vi "QMH_Wait_notifier.vi"(8 "error in (no error)":errorcluster) -> (0 "error out":errorcluster, 2 "Payload":variant, 3 "Message":T1)   [LabVIEW 2021, in "Framework_lib.lvlib"]
uses:
  Framework_lib.lvlib
  QMH_producer_enum.ctl
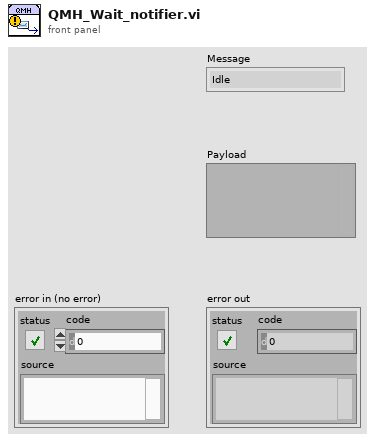
[diagram p1: front panel]
types:
  T1 = typedef "Framework_lib.lvlib/QMH_producer_enum.ctl" = enum16{"Idle", "Initialize", "Shutdown", "ERROR", "Stop", "Start", "Enqueue_frames"}
  T2 = typedef "Framework_lib.lvlib/QMH_references.ctl" = cluster{"Consumer_SUT":refnum<queue>, "Consumer_annotation":refnum<queue>, "compute_results":refnum<queue>, "Notifier":refnum<notifier>}
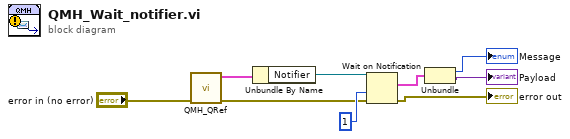
[diagram p0: block diagram]
diagram:
  n1 = call "QMH_QRef.vi"("error in (no error)"="error in (no error)") -> ("error out"=w3:errorcluster, "Cluster Out"=w2:T2)  [unwired: 8 in, 1 out]
  n2 = Unbundle By Name(w2) -> ("Notifier"=w1:refnum<notifier>)
  n3 = Wait on Notification(notifier=w1, timeout in ms (-1)=1, error in (no error)=w3) -> (notification=w7:cluster{"Message":T1, "Payload":variant}, error out=→"error out":errorcluster)  [unwired: 1 in, 2 out]
  n4 = Unbundle(w7) -> ("Message"=→"Message":T1, "Payload"=→"Payload":variant)
